vi "UTF-8 To UTF-16.vi"(8 "error in (no error)":errorcluster, 11 "UTF-8":string) -> (0 "error out":errorcluster, 3 "UTF-16":string)   [LabVIEW 2020, in "G-Audio.lvlib"]
doc: "Converts a UTF-8 encoded string to UTF-16 LE using Windows' MultiByteToWideChar() function.\n\nNote: This function only works on Windows."
uses:
  G-Audio/G-Audio.lvlib
  kernel32.dll
panel:
  # "Force Unicode Text is enabled on this string indicator."
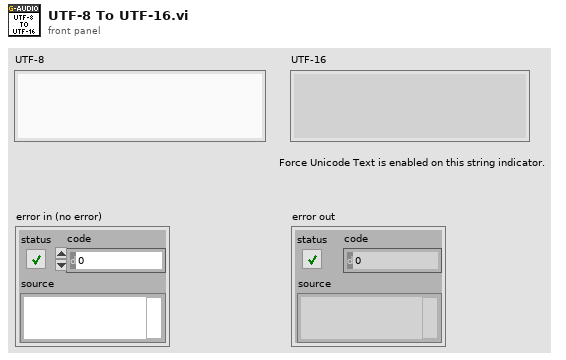
[diagram p1: front panel]
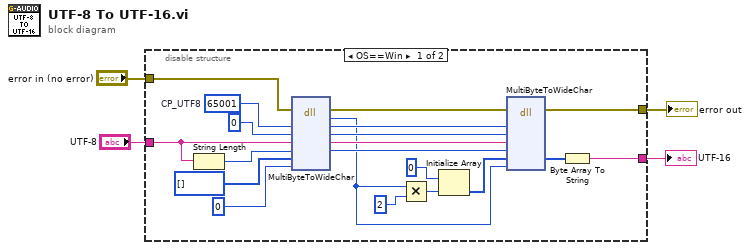
[diagram p0: block diagram]
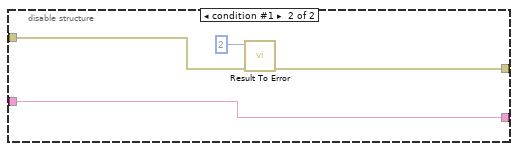
[diagram p2: hidden frame]
diagram:
  n1 = disable-structure shown="OS==Win" {
    disable-tunnel: [w24 w28] -> w4
    disable-tunnel: "UTF-8" -> [w17 w28]
    disable-tunnel: "error in (no error)" -> [w7 w25]
    disable-tunnel: [w5 w26] -> w1
    frame condition #0 (active) {
      w15 = u32 65001  # CP_UTF8
      n2 = String Length(string=w17) -> (length=w18:i32)
      n3 = dll-call lib="kernel32.dll" fn="MultiByteToWideChar"(error in=w7, "codePage"=w15, "dwFlags"=u32 0, "pMultiByteStr"=w17, "cbMultiByte"=w18, "lpWideCharStr"=u8[] [], "cchWideChar"=0) -> (error out=w6:errorcluster, "return type"=w8:i32, "codePage"=w14:u32, "dwFlags"=w13:u32, "pMultiByteStr"=w12:string, "cbMultiByte"=w11:i32)  [unwired: 4 in, 1 out]
      n4 = Multiply(x=w8, y=2) -> (x*y=w10:i32)
      n5 = Initialize Array(u8 0, w10) -> (w22:u8[])
      n6 = dll-call lib="kernel32.dll" fn="MultiByteToWideChar"(error in=w6, "codePage"=w14, "dwFlags"=w13, "pMultiByteStr"=w12, "cbMultiByte"=w11, "lpWideCharStr"=w22, "cchWideChar"=w8) -> (error out=w5:errorcluster, "lpWideCharStr"=w21:u8[])  [unwired: 7 in, 2 out]
      n7 = Byte Array To String(unsigned byte array=w21) -> (string=w24:string)
    }
    frame condition #1 {
      n8 = call "Result To Error.vi"("error in (no error)"=w25, "Result Code"=2) -> ("error out"=w26:errorcluster)  [unwired: 9 in]
    }
  }
  "UTF-16" <- w4
  "error out" <- w1
